vi "DIAdem Process Query Request.vi"(5 "error in (no error)":errorcluster, 7 "DIAdem Queue":T1, 8 "DIAdem Reference":T3) -> (0 "error out":errorcluster, 2 "Results":string, 3 "dup DIAdem Reference":T3)   [LabVIEW 2011]
uses:
  <vilib>/ExportToExcel/DIAdem Reference.ctl
  DIAdem Daemon Queue.ctl
  DIAdem Daemon Script Type.ctl
  Addons/DIAdem/DIAdem.llb/DIAdem String Variable Set.vi
  Addons/DIAdem/DIAdem.llb/DIAdem String Variable Get.vi
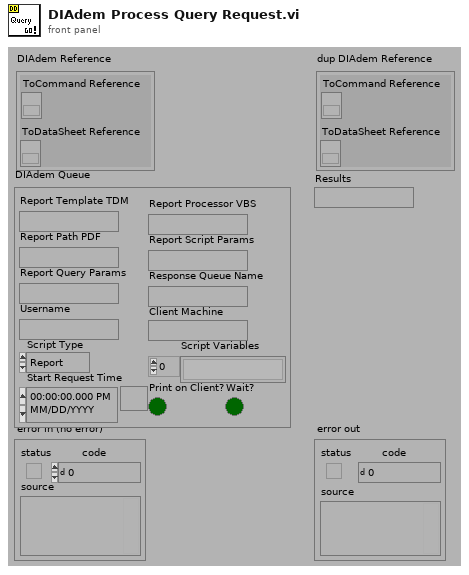
[diagram p1: front panel]
types:
  T1 = typedef "DIAdem Daemon Queue.ctl" = cluster{"Report Template TDM":path, "Report Processor VBS":path, "Report Path PDF":path, "Report Script Params":string, "Username":string, "Script Type":T2, "Report Query Params":string, "Client Machine":string, "Print on Client?":bool, "Response Queue Name":string, "Script Variables":string[], "Start Request Time":timestamp, "Wait?":bool}
  T2 = typedef "DIAdem Daemon Script Type.ctl" = enum16{"Report", "Query", "Script", "Datasheet", "Append", "Restart", "Stop"}
  T3 = typedef "DIAdem Reference.ctl" = cluster{"ToCommand Reference":refnum<k7>, "ToDataSheet Reference":refnum<k7>}
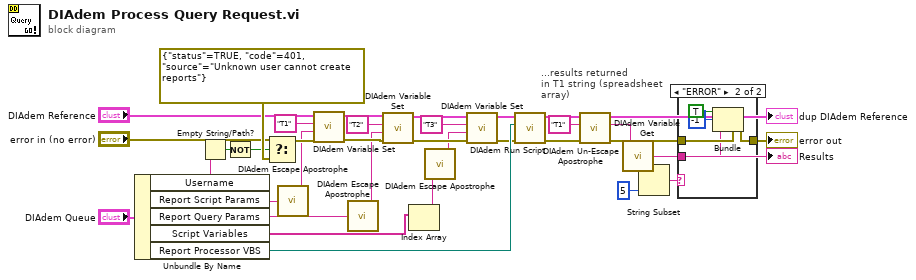
[diagram p0: block diagram]
diagram:
  # "...results returned\nin T1 string (spreadsheet\narray)"
  n1 = Unbundle By Name("DIAdem Queue") -> ("Username"=w30:string, "Report Script Params"=w12:string, "Report Query Params"=w10:string, "Script Variables"=w14:string[], "Report Processor VBS"=w27:path)
  n2 = Empty String/Path?(string/path=w30) -> (empty?=w34:bool)
  n3 = Not(x=w34) -> (.not. x?=w31:bool)
  n4 = Select(t="error in (no error)", s=w31, f=errorcluster {"status"=TRUE, "code"=401, "source"="Unknown user cannot create reports"} ("error in (no error)")) -> (s? t:f=w28:errorcluster)
  n5 = call "DIAdem Escape Apostrophe.vi"("String"=w12) -> ("Escaped String"=w11:string)
  n6 = call-poly "DIAdem Variable Set.vi"("error in (no error)"=w28, "Value"=w11, "Variable Name"="T1", "DIAdem Reference"="DIAdem Reference") -> ("error out"=w21:errorcluster, "DIAdem Reference"=w22:T3)  [unwired: 6 out]
  n7 = call "DIAdem Escape Apostrophe.vi"("String"=w10) -> ("Escaped String"=w9:string)
  n8 = call-poly "DIAdem Variable Set.vi"("error in (no error)"=w21, "Value"=w9, "Variable Name"="T2", "DIAdem Reference"=w22) -> ("error out"=w16:errorcluster, "DIAdem Reference"=w18:T3)  [unwired: 6 out]
  n9 = Index Array(array=w14) -> (element=w8:string)  [unwired: 1 in]
  n10 = call "DIAdem Escape Apostrophe.vi"("String"=w8) -> ("Escaped String"=w7:string)
  n11 = call-poly "DIAdem Variable Set.vi"("error in (no error)"=w16, "Value"=w7, "Variable Name"="T3", "DIAdem Reference"=w18) -> ("error out"=w15:errorcluster, "DIAdem Reference"=w17:T3)  [unwired: 6 out]
  n12 = call "DIAdem Run Script.vi"("error in (no error)"=w15, "script file"=w27, "DIAdem Reference"=w17) -> ("error out"=w13:errorcluster, "DIAdem Reference"=w24:T3)  [unwired: 7 out]
  n13 = call-poly "DIAdem Variable Get.vi"("error in (no error)"=w13, "Variable Name"="T1", "DIAdem Reference"=w24) -> ("error out"=w3:errorcluster, "Value"=w6:string, "DIAdem Reference"=→"dup DIAdem Reference":T3)  [unwired: 6 out]
  n14 = call "DIAdem Un-Escape Apostrophe.vi"("Escaped String"=w6) -> ("String"=w1:string)
  "Results" <- w1
  n15 = String Subset(string=w1, length (rest)=5 ("length (rest)")) -> (substring=w4:string)  [unwired: 1 in]
  n16 = case shown="\"ERROR\"" w4 {
    tunnel: w3 -> [w36 w41]
    tunnel: w1 -> [_ w39]
    tunnel: [w36 w40] -> w2
    frame Default {
    }
    frame "ERROR" {
      n17 = Bundle(cluster=w41, "status"=TRUE, "code"=-1, "source"=w39) -> (w40:errorcluster)
    }
  }
  "error out" <- w2
